vi "Write Sample name.vi"(8 "error in (no error)":errorcluster, 10 "Sample name":string, 11 "Data2D in":refnum<class "Data2D.lvclass">) -> (0 "error out":errorcluster, 3 "Data2D out":refnum<class "Data2D.lvclass">)   [LabVIEW 2014, in "Data2D.lvclass"]
uses:
  Data2D.lvclass
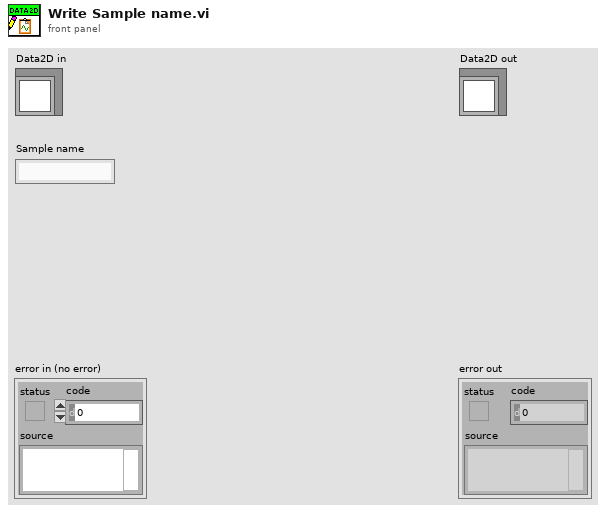
[diagram p1: front panel]
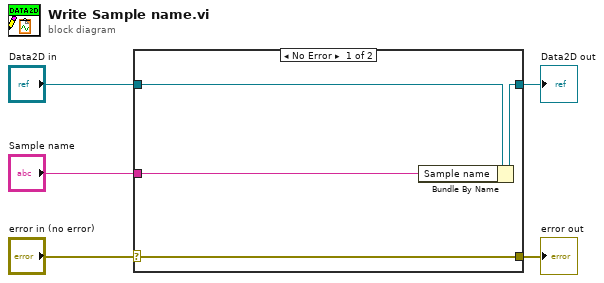
[diagram p0: block diagram]
diagram:
  n1 = case shown="No Error" "error in (no error)" {
    selector: "error in (no error)" -> [w9 w10]
    tunnel: [w9 w10] -> w4
    tunnel: [w7 w11] -> w2
    tunnel: "Data2D in" -> [w8 w11]
    tunnel: "Sample name" -> [w6 _]
    frame No Error {
      n2 = Bundle By Name(cluster=w8, "Sample name"=w6) -> (w7:refnum<class "Data2D.lvclass">)
    }
    frame Error {
    }
  }
  "error out" <- w4
  "Data2D out" <- w2
